vi "TE.vi"(2 "Ctl Refnum":refnum<vi>, 6 "error in (no error)":errorcluster caption="错误输入（无错误）", 7 "目标温度":dbl=80.0, 8 "低温地址":refnum<visa-resource-name>="COM3", 9 "高温":refnum<visa-resource-name> caption="高温地址1", 10 "高温 2":refnum<visa-resource-name> caption="高温地址2", 11 "变温速率1":dbl=3.0) -> (0 "error out":errorcluster caption="错误输出")   [LabVIEW 2017]
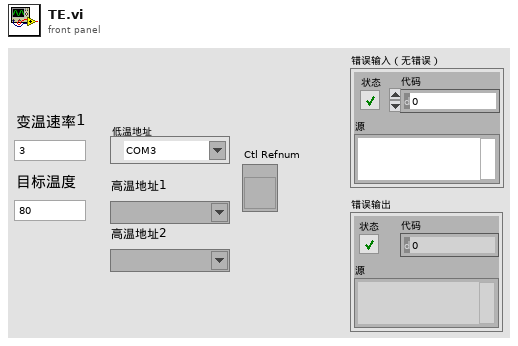
[diagram p1: front panel]
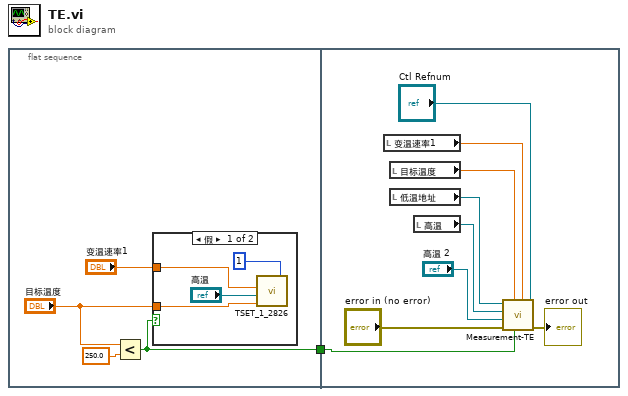
[diagram p0: block diagram]
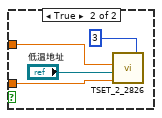
[diagram p2: hidden frame]
diagram:
  n1 = flat-sequence {
    tunnel: [w4] -> w1
    tunnel: w1 -> [w22]
    frame #0 {
      n2 = Less?(x="目标温度", y=250.0) -> (x < y?=w4:bool)
      n3 = case shown="假" w4 {
        tunnel: "变温速率1" -> [w8 w13]
        tunnel: "目标温度" -> [w7 w11]
        frame False {
          n4 = call "TSET_1_2826.vi"("Address No."=i8 1, "T-Ending, C"=w7, "VISA resource name"="高温", "cooling/heating rate, C/min"=w8) -> ()  [unwired: 1 in]
        }
        frame True {
          n5 = call "TSET_2_2826.vi"("Address No."=i8 3, "T-Ending, C"=w11, "VISA resource name"="低温地址", "cooling/heating rate, C/min"=w13) -> ()  [unwired: 1 in]
        }
      }
    }
    frame #1 {
      n6 = local read "变温速率1"() -> (w16:dbl)
      n7 = local read "目标温度"() -> (w17:dbl)
      n8 = local read "低温地址"() -> (w21:refnum<visa-resource-name>)
      n9 = local read "高温"() -> (w15:refnum<visa-resource-name>)
      n10 = call "Measurement-TE.vi"("Ctl Refnum"="Ctl Refnum", "升温速率"=w16, "Boolean"=w22, "目标温度"=w17, "error in (no error)"="error in (no error)", "高温 2"="高温 2", "高温"=w15, "低温地址"=w21) -> ("error out"=→"error out":errorcluster)  [unwired: 3 in]
    }
  }
